vi "Drive Logic Sub (SubVI).vi"(0 "Inputs":T1 {"Kobuki Sensors"."Charger Source" items=["DISCHARGING"=0, "DOCKING_CHARGED"=2, "DOCKING_CHARGING"=6, "ADAPTER_CHARGED"=18, "ADAPTER_CHARGING"=22]; "accelerometer"."z axis (g)" format="%.3f"; "accelerometer"."y axis (g)" format="%.3f"; "accelerometer"."x axis (g)" format="%.3f"}) -> (7 "net angle (deg)":i32, 11 "U-turn Angle":i32, 13 "Soft Left Cliff":bool, 14 "Pause":bool, 15 "U.Turn":bool, 16 "Center":bool, 17 "Hard Right Cliff":bool, 18 "Hard Left Cliff":bool, 19 "Soft Right Cliff":bool)   [LabVIEW 2017]
uses:
  controls/Inputs.ctl
  shared/Accelerometer.ctl
  Kobuki/KobukiSensors.ctl
  Kobuki/Kobuki Bumps and WheelDrops.ctl
  Kobuki/Kobuki Buttons.ctl
panel:
  # "Electrical: charging, battery, OI mode"
  # "Sensors: bump, cliff, button, wheel drop"
  # "Motors:"
  # "Inertia"
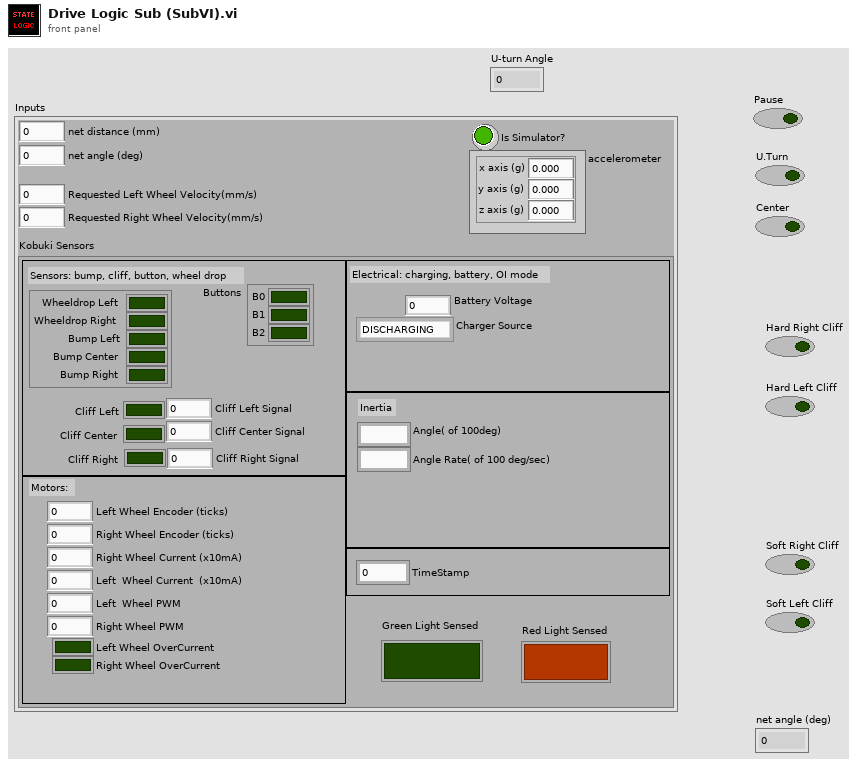
[diagram p1: front panel]
types:
  T1 = typedef "Inputs.ctl" = cluster{"net distance (mm)":i32, "net angle (deg)":i32, "accelerometer":T2, "Is Simulator?":bool, "Kobuki Sensors":T3, "Requested Left Wheel Velocity(mm/s)":i32, "Requested Right Wheel Velocity(mm/s)":i32, "Green Light Sensed":bool, "Red Light Sensed":bool}
  T2 = typedef "Accelerometer.ctl" = cluster{"x axis (g)":dbl, "y axis (g)":dbl, "z axis (g)":dbl}
  T3 = typedef "KobukiSensors.ctl" = cluster{"Bumps + Wheel Drops":T4, "Cliff Left":bool, "Cliff Center":bool, "Cliff Right":bool, "Cliff Left Signal":u16, "Cliff Center Signal":u16, "Cliff Right Signal":u16, "Buttons":T5, "Left Wheel Encoder (ticks)":u16, "Right Wheel Encoder (ticks) ":u16, "Left  Wheel PWM":i8, "Right Wheel PWM":i8, "Left Wheel OverCurrent":bool, "Right Wheel OverCurrent ":bool, "Right Wheel Current (x10mA)":i16, "Left  Wheel Current  (x10mA)":i16, "TimeStamp":u16, "Battery Voltage":dbl, "Angle( of 100deg)":i16, "Angle Rate( of 100 deg/sec)":i16, "Charger Source ":i8}
  T4 = typedef "Kobuki Bumps and WheelDrops.ctl" = cluster{"Wheeldrop Left":bool, "Wheeldrop Right":bool, "Bump Left":bool, "Bump Center":bool, "Bump Right":bool}
  T5 = typedef "Kobuki Buttons.ctl" = cluster{"B0":bool, "B1":bool, "B2":bool}
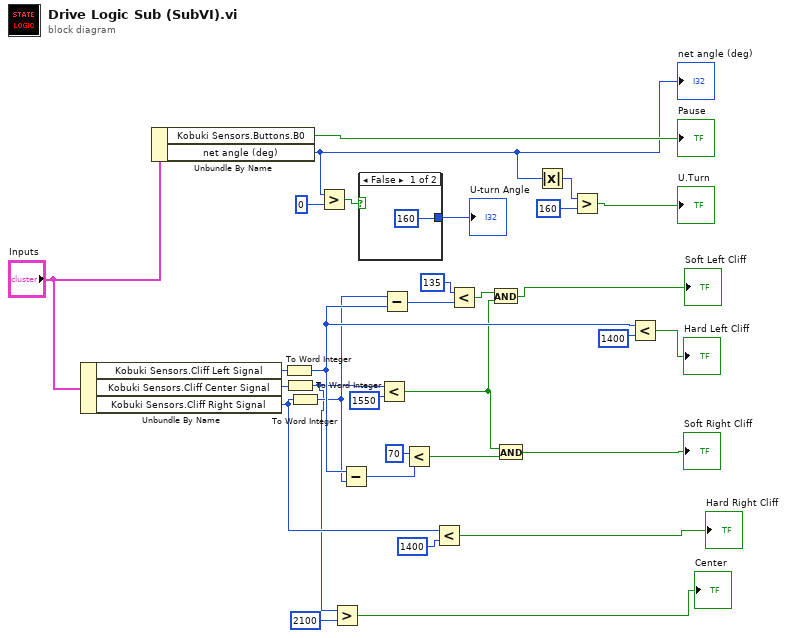
[diagram p0: block diagram]
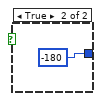
[diagram p2: hidden frame]
diagram:
  n1 = Unbundle By Name("Inputs") -> ("Kobuki Sensors.Cliff Left Signal"=w27:u16, "Kobuki Sensors.Cliff Center Signal"=w28:u16, "Kobuki Sensors.Cliff Right Signal"=w24:u16)
  n2 = Unbundle By Name("Inputs") -> ("Kobuki Sensors.Buttons.B0"=→"Pause":bool, "net angle (deg)"=w6:i32)
  "net angle (deg)" <- w6
  n3 = To Word Integer(number=w27) -> (16bit integer=w26:i16)
  n4 = To Word Integer(number=w28) -> (16bit integer=w3:i16)
  n5 = To Word Integer(number=w24) -> (16bit integer=w25:i16)
  n6 = Greater?(x=w6, y=0) -> (0:w7:bool)
  n7 = Greater?(x=w3, y=i16 2100) -> (0:→"Center":bool)
  n8 = Subtract(x=w26, y=w25) -> (x-y=w19:i16)
  n9 = case shown="False" w7 {
    tunnel: [160 ("y") -180 ("y")] -> w4
    frame False {
    }
    frame True {
    }
  }
  "U-turn Angle" <- w4
  n10 = Less?(x=w3, y=i16 1550) -> (x < y?=w10:bool)
  n11 = Subtract(x=w25, y=w26) -> (x-y=w21:i16)
  n12 = Less?(x=i16 70, y=w19) -> (x < y?=w9:bool)
  n13 = Less?(x=w24, y=u16 1400) -> (x < y?=→"Hard Right Cliff":bool)
  n14 = Less?(x=i16 135, y=w21) -> (x < y?=w23:bool)
  n15 = And(x=w23, y=w10) -> (x .and. y?=→"Soft Left Cliff":bool)
  n16 = And(x=w10, y=w9) -> (x .and. y?=→"Soft Right Cliff":bool)
  n17 = Absolute Value(x=w6) -> (abs(x)=w12:i32)
  n18 = Greater?(x=w12, y=160) -> (0:→"U.Turn":bool)
  n19 = Less?(x=w26, y=i16 1400) -> (x < y?=→"Hard Left Cliff":bool)
